vi "Restart APAR Execution Loop.vi"(8 "error in":errorcluster, 11 "MessageQues":T1) -> (0 "error out":errorcluster)   [LabVIEW 2019]
uses:
  Support/MessageQue/VXM Main Test App/MultipleMessageQues vxm.ctl
  Support/MessageQue/MessageQue.ctl
  Support/MessageQue/MessageCluster.ctl
  Support/MessageQue/MessageQue.lvlib
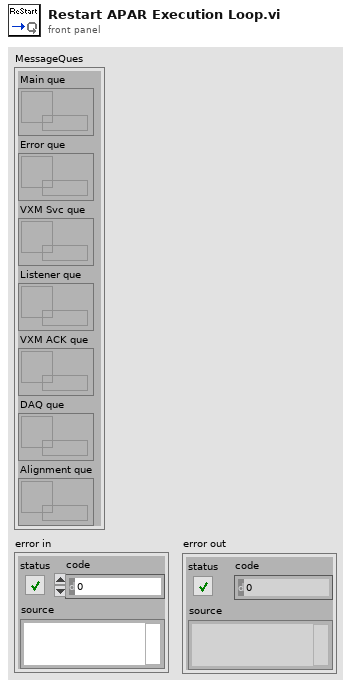
[diagram p1: front panel]
types:
  T1 = typedef "MultipleMessageQues vxm.ctl" = cluster{"Main que":T2, "Error que":T2, "VXM Svc que":T2, "Listener que":T2, "VXM ACK que":T2, "DAQ que":T2, "Alignment que":T2}
  T2 = typedef "MessageQue.lvlib/MessageQue.ctl" = refnum<queue>
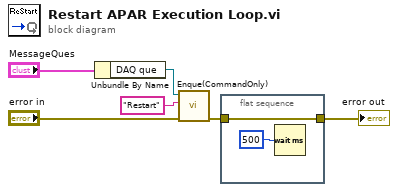
[diagram p0: block diagram]
diagram:
  n1 = Unbundle By Name("MessageQues") -> ("DAQ que"=w4:T2)
  n2 = call "Enque(CommandOnly).vi"("error in"="error in", "Message Command"="Restart", "Message que"=w4) -> ("error out"=w2:errorcluster)  [unwired: 7 in, 1 out]
  n3 = flat-sequence {
    tunnel: w2 -> [w7]
    tunnel: [w7] -> w1
    frame #0 {
      n4 = Wait (ms)(milliseconds to wait=u32 500) -> ()  [unwired: 1 out]
    }
  }
  "error out" <- w1
